vi "PIM Compare and Coerce Stimulus.vi"(6 "Driver Ref (null)":T1, 8 "error in (no error)":errorcluster, 10 "Flat TestSetDef Params":string, 11 "PIM Test Parameters":T2={"Stimulus"={"C1 Pwr dBm"=0.0, "C2 Pwr dBm"=0.0, "Power Units"=enum."dBm", "Meas Type"=enum."Time", "C1 Freq MHz"=0.0, "C2 Freq MHz"=0.0, "Swept Freq Step"=0}, "Measure"={"IM Order"=0, "Direction"=0, "Averaging"=1, "ALC ON?"=TRUE, "Peak Hold?"=TRUE, "Peak last N"=1, "Ref Level dBm"=-100.0, "Ref Units"=enum."dBm", "Num Samples"=1, "Sample units"=enum."Sample(s)", "Update Rate (s)"=0.0, "DUT PORT"=enum."Port 1", "Percent (%)"=100}, "Display"={"Power Scale"={"yRange_min"=0, "yRange_max"=0}, "xRange_span"=5}} {"Stimulus"."Swept Freq Step" items=[".2", ".4", "1.0", "2.0"]; "Measure"."Averaging" items=["None", "Minimum", "Normal", "High", "Maximum"]; "Measure"."Direction" items=["Reverse", "Forward", "Auxiliary"]; "Measure"."IM Order" items=["3rd", "5th", "7th", "9th", "11th", "13th", "15th", "17th", "19th", "21st", "23rd", "25th", "27th", "29th", "31st", "33rd"]}) -> (0 "error out":errorcluster, 3 "Corrected Test Params":T2={"Stimulus"={"C1 Pwr dBm"=0.0, "C2 Pwr dBm"=0.0, "Power Units"=enum."dBm", "Meas Type"=enum."Time", "C1 Freq MHz"=0.0, "C2 Freq MHz"=0.0, "Swept Freq Step"=0}, "Measure"={"IM Order"=0, "Direction"=0, "Averaging"=1, "ALC ON?"=TRUE, "Peak Hold?"=TRUE, "Peak last N"=1, "Ref Level dBm"=-100.0, "Ref Units"=enum."dBm", "Num Samples"=1, "Sample units"=enum."Sample(s)", "Update Rate (s)"=0.0, "DUT PORT"=enum."Port 1", "Percent (%)"=100}, "Display"={"Power Scale"={"yRange_min"=0, "yRange_max"=0}, "xRange_span"=5}} {"Stimulus"."Swept Freq Step" items=[".2", ".4", "1.0", "2.0"]; "Measure"."Averaging" items=["None", "Minimum", "Normal", "High", "Maximum"]; "Measure"."Direction" items=["Reverse", "Forward", "Auxiliary"]; "Measure"."IM Order" items=["3rd", "5th", "7th", "9th", "11th", "13th", "15th", "17th", "19th", "21st", "23rd", "25th", "27th", "29th", "31st", "33rd"]}, 4 "TestSetDef":T12={"General"={"ID"=0, "Model"="", "Dual Port?"=FALSE, "Options"="", "Options"={"E"=FALSE, "K"=FALSE, "H"=FALSE, "W"=FALSE, "F"=FALSE}, "Cal File"=path ""}, "Receiver"={"Fstart, MHz"=0.0, "Fstop MHz"=0.0, "Fstep MHz"=0.0, "IF, MHz"=0.0}, "RX Band"={"Fstart, MHz"=0.0, "Fstop MHz"=0.0}, "TX 1"={"Fstart, MHz"=0.0, "Fstop MHz"=0.0, "Pmax, dBm"=0.0, "Pstep, dB"=0.0}, "TX 2"={"Fstart, MHz"=0.0, "Fstop MHz"=0.0, "Pmax, dBm"=0.0, "Pstep, dB"=0.0}, "Low-side?"=TRUE})   [LabVIEW 2011]
uses:
  BPIMCore/HW IO/Test Set Definition.ctl
  TypeDefs/PIM Test Parameters.ctl
  TypeDefs/PIM Stimulus Parameters.ctl
  BPIMCore/HW IO/PIM Sweep Step Size.ctl
  TypeDefs/PIM Measurement Parameters.ctl
  BPIMCore/HW IO/IMOrder.ctl
  BPIMCore/HW IO/MeasMode.ctl
  BPIMCore/HW IO/HW Averaging.ctl
  TypeDefs/PIM Meas Units.ctl
  BPIMCore/HW IO/DUTport.ctl
  TypeDefs/PIM Display Parameters.ctl
  drivers/PIM/PIM Driver Ref.ctl
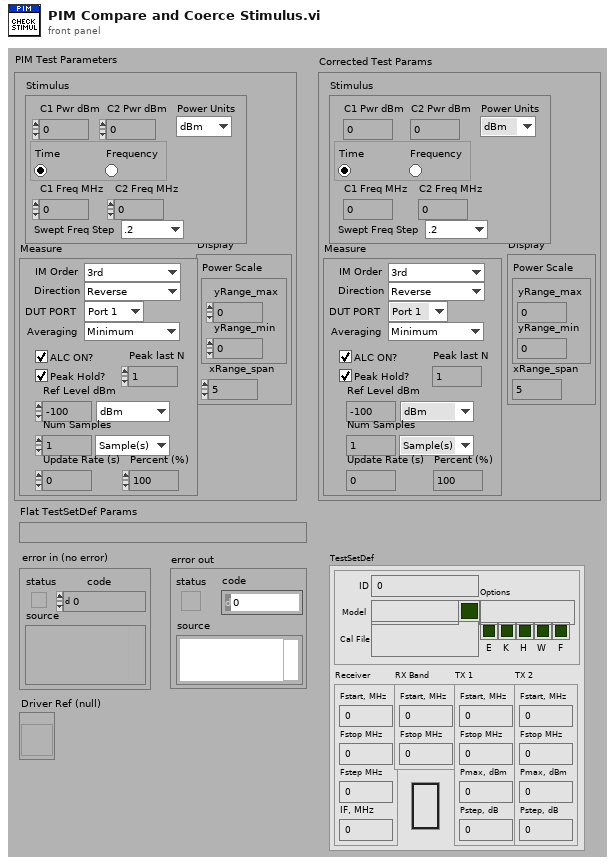
[diagram p1: front panel]
types:
  T1 = typedef "PIM Driver Ref.ctl" = refnum<vi>
  T2 = typedef "PIM Test Parameters.ctl" = cluster{"Stimulus":T3, "Measure":T5, "Display":T11}
  T3 = typedef "PIM Stimulus Parameters.ctl" = cluster{"C1 Pwr dBm":dbl, "C2 Pwr dBm":dbl, "Power Units":enum16{"dBm", "Watts"}, "Meas Type":enum32{"Time", "Frequency"}, "C1 Freq MHz":dbl, "C2 Freq MHz":dbl, "Swept Freq Step":T4}
  T4 = typedef "PIM Sweep Step Size.ctl" = u16
  T5 = typedef "PIM Measurement Parameters.ctl" = cluster{"IM Order":T6, "Direction":T7, "Averaging":T8, "ALC ON?":bool, "Peak Hold?":bool, "Peak last N":u32, "Ref Level dBm":dbl, "Ref Units":enum16{"dBm", "dBc"}, "Num Samples":u32, "Sample units":T9, "Update Rate (s)":dbl, "DUT PORT":T10, "Percent (%)":u8}
  T6 = typedef "IMOrder.ctl" = u8
  T7 = typedef "MeasMode.ctl" = u16
  T8 = typedef "HW Averaging.ctl" = u16
  T9 = typedef "PIM Meas Units.ctl" = enum16{"Sample(s)", "Second(s)", "Sweep(s)"}
  T10 = typedef "DUTport.ctl" = enum16{"Port 1", "Port 2"}
  T11 = typedef "PIM Display Parameters.ctl" = cluster{"Power Scale":cluster{"yRange_min":i32, "yRange_max":i32}, "xRange_span":u32}
  T12 = typedef "Test Set Definition.ctl" = cluster{"General":cluster{"ID":u32, "Model":string, "Dual Port?":bool, "Options":string, "Options":cluster{"E":bool, "K":bool, "H":bool, "W":bool, "F":bool}, "Cal File":path}, "Receiver":cluster{"Fstart, MHz":dbl, "Fstop MHz":dbl, "Fstep MHz":dbl, "IF, MHz":dbl}, "RX Band":cluster{"Fstart, MHz":dbl, "Fstop MHz":dbl}, "TX 1":cluster{"Fstart, MHz":dbl, "Fstop MHz":dbl, "Pmax, dBm":dbl, "Pstep, dB":dbl}, "TX 2":cluster{"Fstart, MHz":dbl, "Fstop MHz":dbl, "Pmax, dBm":dbl, "Pstep, dB":dbl}, "Low-side?":bool}
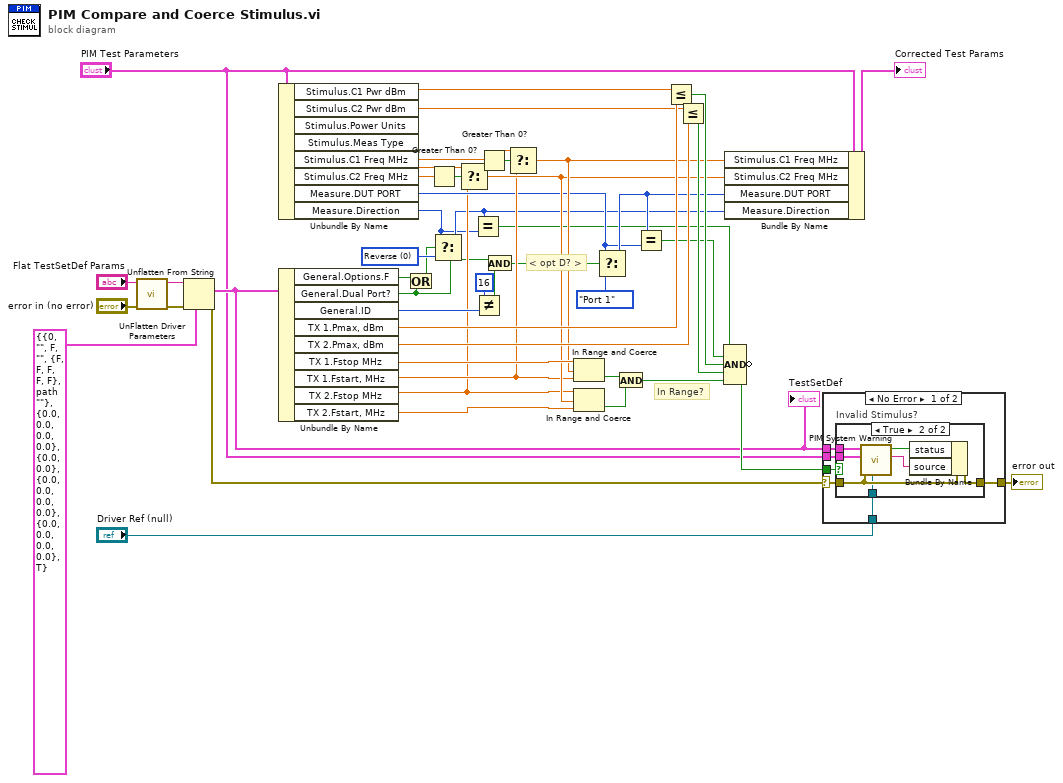
[diagram p0: block diagram]
diagram:
  w5 = T7 0 items=["Reverse", "Forward", "Auxiliary"] ("Measure.Direction")
  # "< opt D? >"
  # "In Range?"
  n1 = call "UnFlatten Driver Parameters.vi"("error in (no error)"="error in (no error)", "Flattened Driver Parameters with Version (\"\")"="Flat TestSetDef Params") -> ("error out"=w42:errorcluster, "Flat Driver Parameters"=w44:string)  [unwired: 4 out]
  n2 = Unflatten From String(type=T12 {"General"={"ID"=0, "Model"="", "Dual Port?"=FALSE, "Options"="", "Options"={"E"=FALSE, "K"=FALSE, "H"=FALSE, "W"=FALSE, "F"=FALSE}, "Cal File"=path ""}, "Receiver"={"Fstart, MHz"=0.0, "Fstop MHz"=0.0, "Fstep MHz"=0.0, "IF, MHz"=0.0}, "RX Band"={"Fstart, MHz"=0.0, "Fstop MHz"=0.0}, "TX 1"={"Fstart, MHz"=0.0, "Fstop MHz"=0.0, "Pmax, dBm"=0.0, "Pstep, dB"=0.0}, "TX 2"={"Fstart, MHz"=0.0, "Fstop MHz"=0.0, "Pmax, dBm"=0.0, "Pstep, dB"=0.0}, "Low-side?"=TRUE} ("Test Set Definition"), binary string=w44, error in (no error)=w42) -> (value=w40:T12, error out=w38:errorcluster)  [unwired: 3 out]
  "TestSetDef" <- w40
  n3 = Unbundle By Name("PIM Test Parameters") -> ("Stimulus.C1 Pwr dBm"=w27:dbl, "Stimulus.C2 Pwr dBm"=w26:dbl, "Stimulus.C1 Freq MHz"=w25:dbl, "Stimulus.C2 Freq MHz"=w21:dbl, "Measure.DUT PORT"=w11:T10, "Measure.Direction"=w2:T7)  [unwired: 2 out]
  n4 = Unbundle By Name(w40) -> ("General.Options.F"=w7:bool, "General.Dual Port?"=w6:bool, "General.ID"=w13:u32, "TX 1.Pmax, dBm"=w34:dbl, "TX 2.Pmax, dBm"=w33:dbl, "TX 1.Fstop MHz"=w35:dbl, "TX 1.Fstart, MHz"=w24:dbl, "TX 2.Fstop MHz"=w9:dbl, "TX 2.Fstart, MHz"=w20:dbl)
  n5 = Or(x=w7, y=w6) -> (x .or. y?=w4:bool)
  n6 = Greater Than 0?(x=w21) -> (x > 0?=w22:bool)
  n7 = Select(t=w2, s=w4, f=w5) -> (s? t:f=w3:T7)
  n8 = Select(t=w21, s=w22, f=w9) -> (s? t:f=w28:dbl)
  n9 = Equal?(x=w3, y=w2) -> (x = y?=w1:bool)
  n10 = Not Equal?(x=16 ("y"), y=w13) -> (x != y?=w17:bool)
  n11 = Greater Than 0?(x=w25) -> (x > 0?=w23:bool)
  n12 = And(x=w6, y=w17) -> (x .and. y?=w15:bool)
  n13 = Select(t=w25, s=w23, f=w24) -> (s? t:f=w29:dbl)
  n14 = In Range and Coerce(upper limit=w35, x=w29, lower limit=w24) -> (In Range?=w19:bool)  [unwired: 1 out]
  n15 = In Range and Coerce(upper limit=w9, x=w28, lower limit=w20) -> (In Range?=w18:bool)  [unwired: 1 out]
  n16 = Select(t=w11, s=w15, f=DUTport."Port 1" ("Measure.DUT PORT")) -> (s? t:f=w12:T10)
  n17 = And(x=w19, y=w18) -> (x .and. y?=w32:bool)
  n18 = Equal?(x=w12, y=w11) -> (x = y?=w10:bool)
  n19 = Less Or Equal?(x=w27, y=w34) -> (x <= y?=w31:bool)
  n20 = Less Or Equal?(x=w26, y=w33) -> (x <= y?=w30:bool)
  n21 = Compound Arithmetic op=AND(w1, w10, w31, w30, w32) -> (invert w41:bool)
  n22 = Bundle By Name(cluster="PIM Test Parameters", "Stimulus.C1 Freq MHz"=w29, "Stimulus.C2 Freq MHz"=w28, "Measure.DUT PORT"=w12, "Measure.Direction"=w3) -> (→"Corrected Test Params":T2)
  n23 = case shown="No Error" w38 {
    selector: w38 -> [w48 w61]
    tunnel: w41 -> [w52 _]
    tunnel: w40 -> [w51 _]
    tunnel: [w50 w61] -> w39
    tunnel: "PIM Test Parameters" -> [w49 _]
    tunnel: "Driver Ref (null)" -> [w47 _]
    frame No Error {
      n24 = case "Invalid Stimulus?" shown="True" w52 {
        tunnel: w51 -> [_ w60]
        tunnel: w49 -> [_ w59]
        tunnel: w48 -> [w53 w55]
        tunnel: [w53 w58] -> w50
        tunnel: w47 -> [_ w54]
        frame False {
        }
        frame True {
          n25 = call "PIM System Warning.vi"("Driver Ref (null)"=w54, "error in (no error)"=w55, "PIM Test Parameters"=w59, "TestSetDef"=w60) -> ("Message (\"\")"=w56:string, "Abort?"=w57:bool)  [unwired: 6 out]
          n26 = Bundle By Name(cluster=w55, "status"=w57, "source"=w56) -> (w58:errorcluster)
        }
      }
    }
    frame Error {
      # "If we're in an error state, pass\nthe driver error through to the\nclient machine."
    }
  }
  "error out" <- w39
